vi "Analyse Images.vi"(6 "Analysis Mode":T1=enum."Full Run", 8 "error in (no error)":errorcluster, 9 "Local Data in":T2, 10 "UI Refs":T9, 11 "TCP Network Connection in":refnum<k5>) -> (0 "error out":errorcluster, 3 "TCP Network Connection out":refnum<k5>)   [LabVIEW 2024]
uses:
  Controls/RVHR - UI Refs.ctl
  Controls/RVHR - Local Data.ctl
  Controls/Test Cluster.ctl
  Controls/Excluded Information.ctl
  Controls/Language.ctl
  Controls/Device_Type.ctl
  <vilib>/Utility/miscctls.llb/LVRectTypeDef.ctl
  <vilib>/Utility/miscctls.llb/LVBoundsTypeDef.ctl
  Controls/RVHR - Analysis Mode.ctl
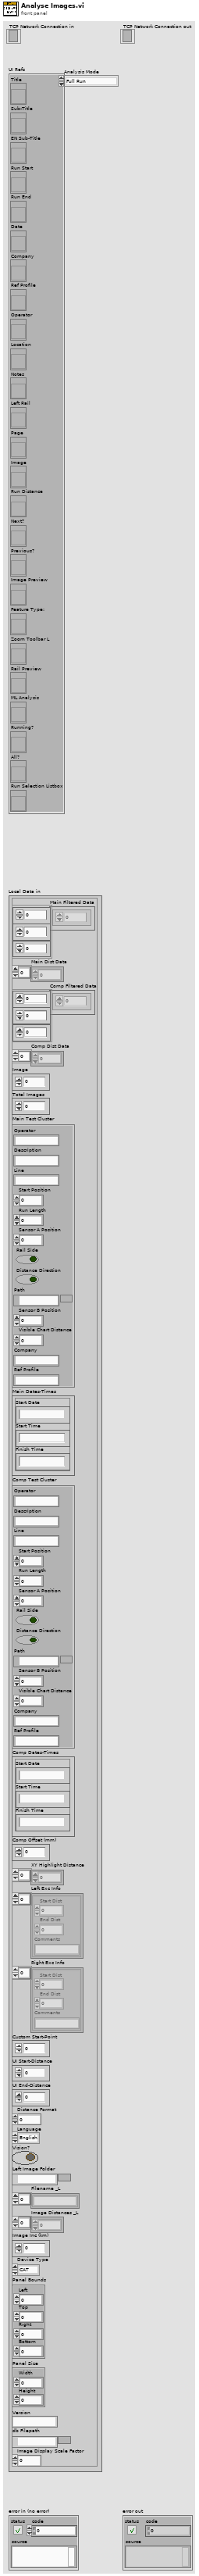
[diagram p1: front panel]
types:
  T1 = typedef "RVHR - Analysis Mode.ctl" = enum16{"Current Images", "Full Run"}
  T2 = typedef "RVHR - Local Data.ctl" = cluster{"Main Filtered Data":dbl[][][], "Main Dist Data":dbl[], "Comp Filtered Data":dbl[][][], "Comp Dist Data":dbl[], "Image":u16, "Total Images":u16, "Main Test Cluster":T3, "Main Dates-Times":cluster{"Start Date":string, "Start Time":string, "Finish Time":string}, "Comp Test Cluster":T3, "Comp Dates-Times":cluster{"Start Date":string, "Start Time":string, "Finish Time":string}, "Comp Offset (mm)":i64, "XY Highlight Distance":dbl[], "Left Exc Info":T4[], "Right Exc Info":T4[], "Custom Start-Point":dbl, "UI Start-Distance":dbl, "UI End-Distance":dbl, "Distance Format":u8, "Language":T5, "Vision?":bool, "Left Image Folder":path, "Filename _L":string[], "Image Distances _L":dbl[], "Image Inc (km)":dbl, "Device Type":T6, "Panel Bounds":T7, "Panel Size":T8, "Version":string, "db Filepath":path, "Image Display Scale Factor":dbl}
  T3 = typedef "Test Cluster.ctl" = cluster{"Operator":string, "Description":string, "Line":string, "Start Position":dbl, "Run Length":dbl, "Sensor A Position":dbl, "Rail Side":bool, "Distance Direction":bool, "Path":path, "Sensor B Position":dbl, "Visible Chart Distance":dbl, "Company":string, "Ref Profile":string}
  T4 = typedef "Excluded Information.ctl" = cluster{"Start Dist":dbl, "End Dist":dbl, "Comments":string}
  T5 = typedef "Language.ctl" = enum16{"English", "Chinese", "German"}
  T6 = typedef "Device_Type.ctl" = enum16{"CAT", "Bi-CAT", "YRCA", "RCA", "RV-HR", "TV-HR"}
  T7 = typedef "LVRectTypeDef.ctl" = cluster{"Left":i16, "Top":i16, "Right":i16, "Bottom":i16}
  T8 = typedef "LVBoundsTypeDef.ctl" = cluster{"Width":u32, "Height":u32}
  T9 = typedef "RVHR - UI Refs.ctl" = cluster{"Title":refnum<vi>, "Sub-Title":refnum<vi>, "EN Sub-Title":refnum<vi>, "Run Start":refnum<vi>, "Run End":refnum<vi>, "Date":refnum<vi>, "Company":refnum<vi>, "Ref Profile":refnum<vi>, "Operator":refnum<vi>, "Location":refnum<vi>, "Notes":refnum<vi>, "Left Rail":refnum<vi>, "Page":refnum<vi>, "Image":refnum<vi>, "Run Distance":refnum<vi>, "Next?":refnum<vi>, "Previous?":refnum<vi>, "Image Preview":refnum<vi>, "Feature Type:":refnum<vi>, "Zoom Toolbar L":refnum<vi>, "Rail Preview":refnum<vi>, "ML Analysis":refnum<vi>, "Running?":refnum<vi>, "All?":refnum<vi>, "Run Selection Listbox":refnum<vi>}
  T10 = enum8{"Enabled", "Disabled", "Disabled and Grayed Out"}
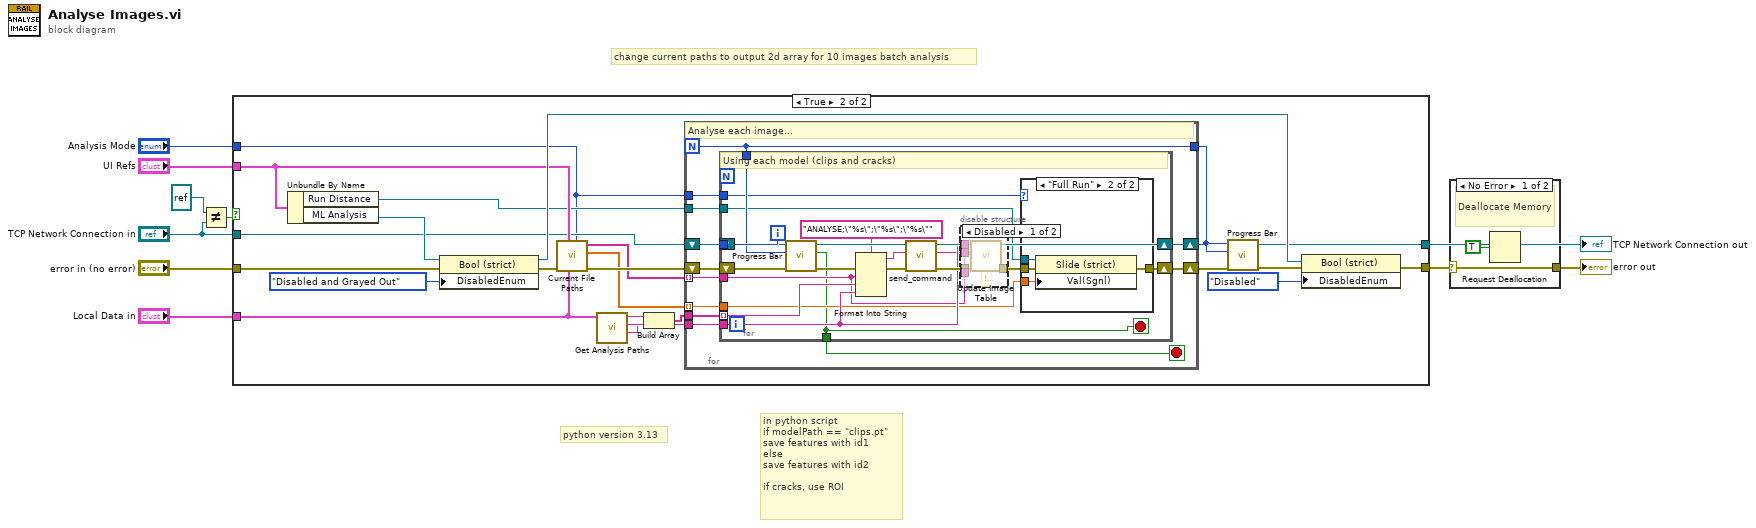
[diagram p0: block diagram]
diagram:
  # "change current paths to output 2d array for 10 images batch analysis"
  # "python version 3.13"
  # "in python script\nif modelPath == \"clips.pt\"\nsave features with id1\nelse\nsave features with id2\n\nif cracks, use ROI"
  n1 = Not Equal?(x=refnum<k5> refnum, y="TCP Network Connection in") -> (x != y?=w5:bool)
  n2 = case shown="True" w5 {
    tunnel: [w12 w33] -> w2
    tunnel: "UI Refs" -> [_ w31]
    tunnel: "error in (no error)" -> [w12 w29]
    tunnel: "Local Data in" -> [_ w25]
    tunnel: "TCP Network Connection in" -> [w11 w21]
    tunnel: [w11 w20] -> w7
    tunnel: "Analysis Mode" -> [_ w17]
    frame False {
    }
    frame True {
      n3 = Unbundle By Name(w31) -> ("Run Distance"=w19:refnum<vi>, "ML Analysis"=w27:refnum<vi>)
      n4 = property class="Bool (strict)"(reference=w27, error in=w29, "DisabledEnum"=T10."Disabled and Grayed Out" ("Disabled")) -> (reference out=w32:refnum<vi>, error out=w30:errorcluster)
      n5 = call "Current File Paths.vi"("Analysis Mode"=w17, "Local Data in"=w25, "UI Refs"=w31, "error in (no error)"=w30) -> ("error out"=w24:errorcluster, "Distances"=w18:dbl[], "Tags"=w23:string[])  [unwired: 5 in]
      n6 = call "Get Analysis Paths.vi"("Local Data in"=w25) -> ("CrackModelPath"=w14:string, "DBPath"=w22:string, "ClipModelPath"=w15:string)  [unwired: 8 in]
      n7 = Build Array(w15, w14) -> (w13:string[])
      n8 = for {
        N -> [w43]
        shift-right: [w39] -> w16
        shift-left: w24 -> [w44]
        shift-right: [w47] -> w20
        shift-left: w21 -> [w48]
        tunnel: w13 -> [w46]
        tunnel: w22 -> [w42]
        tunnel: w23 -> [w41] mode=indexing
        tunnel: [w43] -> w35
        tunnel: w19 -> [w38]
        tunnel: w18 -> [w37] mode=indexing
        tunnel: w17 -> [w36]
        i -> [w45]
        stop <- w40 stop-if-true
        # "Analyse each image..."
        n9 = for {
          tunnel: w46 -> [w64] mode=indexing
          tunnel: w45 -> [w63]
          tunnel: w43 -> [w60]
          tunnel: w42 -> [w57]
          tunnel: w41 -> [w56]
          tunnel: [w49] -> w40
          tunnel: w38 -> [w52]
          tunnel: w37 -> [w51]
          tunnel: w36 -> [w50]
          shift-right: [w67] -> w47
          shift-left: w48 -> [w68]
          shift-right: [w53] -> w39
          shift-left: w44 -> [w62]
          stop <- w49 stop-if-true
          # "Using each model (clips and cracks)"
          n10 = call "Progress Bar.vi"("error in"=w62, "N"=w60, "i"=w63) -> ("error out"=w61:errorcluster, "Stop?"=w49:bool)  [unwired: 6 in, 1 out]
          n11 = Format Into String(format string="ANALYSE;\"%s\";\"%s\";\"%s\"" ("replace string (\"\")"), error in=w61, w56, w64, w57) -> (resulting string=w54:string, error out=w65:errorcluster)  [unwired: 1 in]
          n12 = call "send_command.vi"("error in (no error)"=w65, "command"=w54, "connection ID"=w68) -> ("error out"=w59:errorcluster, "response"=w55:string, "connection ID out"=w67:refnum<k5>)  [unwired: 6 in]
          n13 = disable-structure shown="Disabled" {
            disable-tunnel: w59 -> [w73 w74]
            disable-tunnel: [w72 w74] -> w58
            disable-tunnel: w57 -> [w71 _]
            disable-tunnel: w56 -> [w70 _]
            disable-tunnel: w55 -> [w69 _]
            frame Disabled {
              # "!!"
              n14 = call "Update Image Table.vi"("error in (no error)"=w73, "Image Path"=w70, "response"=w69, "DB Path"=w71) -> ("error out"=w72:errorcluster)  [unwired: 7 in]
            }
            frame Enabled {
            }
          }
          n15 = case shown="\"Full Run\"" w50 {
            tunnel: w58 -> [w75 w79]
            tunnel: [w75 w78] -> w53
            tunnel: w52 -> [_ w77]
            tunnel: w51 -> [_ w76]
            frame "Current Images", Default {
            }
            frame "Full Run" {
              n16 = property class="Slide (strict)"(reference=w77, error in=w79, "Val(Sgnl)"=w76) -> (error out=w78:errorcluster)  [unwired: 1 out]
            }
          }
        }
      }
      n17 = call "Progress Bar.vi"("error in"=w16, "N"=w35, "i"=w35) -> ("error out"=w34:errorcluster)  [unwired: 6 in, 2 out]
      n18 = property class="Bool (strict)"(reference=w32, error in=w34, "DisabledEnum"=T10."Disabled" ("Disabled")) -> (error out=w33:errorcluster)  [unwired: 1 out]
    }
  }
  "TCP Network Connection out" <- w7
  n19 = case shown="No Error" w2 {
    selector: w2 -> [w80 w82]
    tunnel: [w80 w82] -> w1
    frame No Error {
      # "Deallocate Memory"
      n20 = Request Deallocation(TRUE ("flag")) -> ()
    }
    frame Error {
    }
  }
  "error out" <- w1
